vi "TurnForTime.vi"(8 "error in":errorcluster, 10 "Time (ms)":u32, 11 "Speed/Direction":dbl) -> (0 "error out":errorcluster)   [LabVIEW 2016]
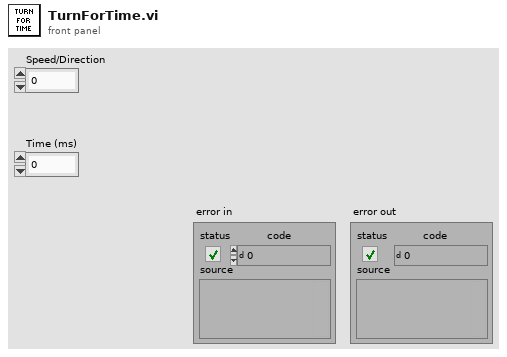
[diagram p1: front panel]
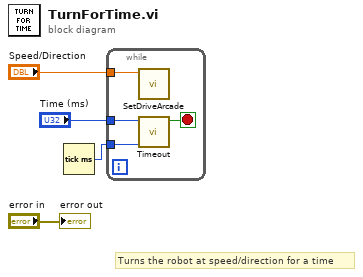
[diagram p0: block diagram]
diagram:
  # "Turns the robot at speed/direction for a time"
  n1 = Tick Count (ms)() -> (millisecond timer value=w2:u32)
  n2 = while {
    tunnel: "Time (ms)" -> [w8]
    tunnel: "Speed/Direction" -> [w5]
    tunnel: w2 -> [w6]
    stop <- w7 stop-if-true
    n3 = call "SetDriveArcade.vi"("Turn"=w5) -> ()  [unwired: 10 in, 1 out]
    n4 = call "Timeout.vi"("Start Time In"=w6, "Time Limit"=w8) -> ("Timeout"=w7:bool)  [unwired: 8 in, 1 out]
  }
  "error out" <- "error in"
